vi "Get Connection ID.vi"(8 "error in (no error)":errorcluster, 11 "Connection Reference In":refnum<data-value>) -> (0 "error out":errorcluster, 2 "ID":string, 3 "Connection Reference Out":refnum<data-value>)   [LabVIEW 2019, in "Connection Reference.lvlib" / "Connection Reference.lvclass"]
uses:
  <vilib>/gpm_packages/@cs/Network-interface/Source/Connection Reference/Connection Reference/Connection Reference.lvclass
  <vilib>/gpm_packages/@cs/Network-interface/Source/Connection Reference/Connection Reference/Connection Reference.lvclass/Connection Reference.ctl
  <vilib>/gpm_packages/@cs/Network-interface/Source/Connection Reference/IConnection/IConnection.lvclass
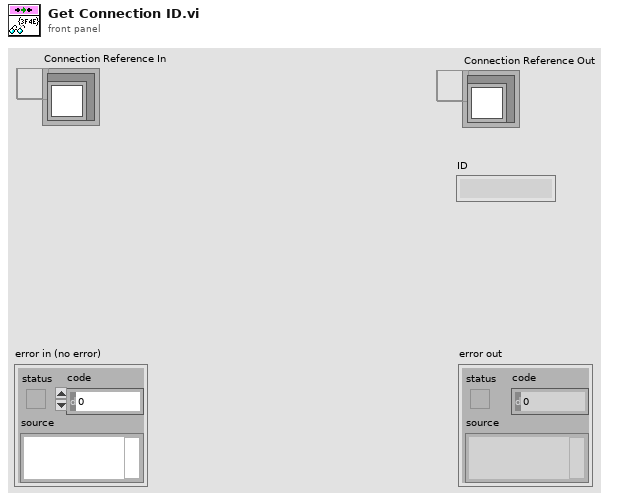
[diagram p1: front panel]
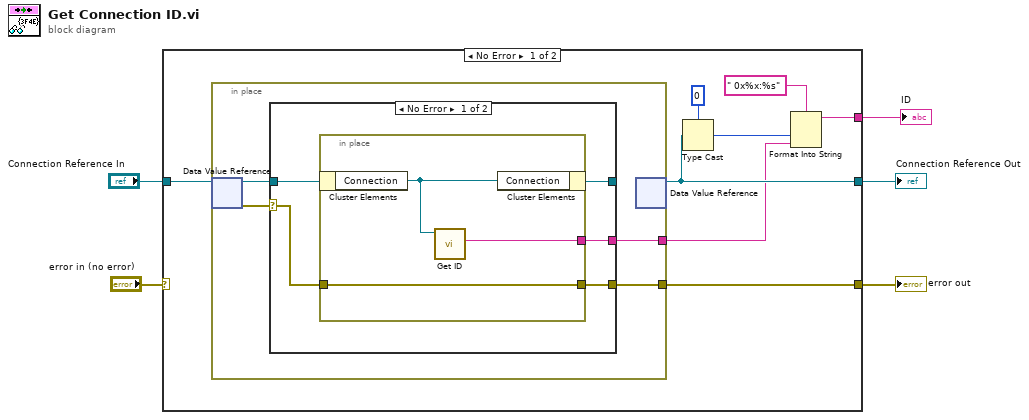
[diagram p0: block diagram]
diagram:
  n1 = case shown="No Error" "error in (no error)" {
    selector: "error in (no error)" -> [_ w28]
    tunnel: "Connection Reference In" -> [w13 w29]
    tunnel: [w8 w29] -> w4
    tunnel: [w12 w28] -> w2
    tunnel: [w10 _] -> w1
    frame No Error {
      n2 = in-place {
        in-place-border: [w15] -> w12
        in-place-border: [w14] -> w6
        n3 = in-place-dvr #1(w13) -> (w17:refnum<class "Connection Reference.lvclass">, w16:errorcluster)
        n4 = case shown="No Error" w16 {
          selector: w16 -> [w19 w26]
          tunnel: w17 -> [w22 w27]
          tunnel: [w21 w27] -> _
          tunnel: [w20 w26] -> w15
          tunnel: [w18 _] -> w14
          frame No Error {
            n5 = in-place {
              in-place-border: [w24] -> w20
              in-place-border: w19 -> [w24]
              in-place-border: [w23] -> w18
              n6 = in-place-cluster #2(w22) -> ("Connection"=w25:refnum<class "IConnection.lvclass">)
              n7 = call-dynamic "Get ID.vi"("IConnection in"=w25) -> ("ID"=w23:string)  [unwired: 10 in]
              n8 = in-place-cluster #2("Connection"=w25) -> (w21:refnum<class "Connection Reference.lvclass">)
            }
          }
          frame Error {
            # "#todo add useful error here"
          }
        }
        n9 = in-place-dvr #1() -> (w8:refnum<data-value>)  [unwired: 1 in, 1 out]
      }
      n10 = Type Cast(type=0, x=w8) -> (*(type *) &x=w11:i32)
      n11 = Format Into String(format string=" 0x%x:%s", w11, w6) -> (resulting string=w10:string)  [unwired: 2 in, 1 out]
    }
    frame Error {
    }
  }
  "error out" <- w2
  "Connection Reference Out" <- w4
  "ID" <- w1
